vi "9T position.vi"(11 "Instrument":T1={"325 Resource "="GPIB0::13::INSTR", "Input (0:A) 325"=0, "Heater Output (1:1) 325"=1, "340 Resource"="GPIB0::14::INSTR", "Input (0:A) 340"=0, "Loop (0: 1)"=0, "Input (0:B) 340"=1, "Loop (1: 1)"=0, "340 Status"=refnum, "Instrument Type"=enum."PPMS-Rotate", "quantum design"=refnum, "semaphore 325"=refnum, "TCP master instance"=refnum, "M24C Resource"="GPIB0::24::INSTR", "4G supply"="GPIB0::24::INSTR", "Temp Status 24C"=refnum, "Temp"=refnum, "9T信号"=refnum, "limit"={"Field limit"=0.0, "Field rate limit"=0.0, "Temp limit"=0.0, "Temp low limit"=0.0, "Temp rate limit "=0.0}, "4g supply status"=refnum, "vi路径"="", "in-plane"="", "out-plane"="", "in-plane signal"=FALSE, "out-plane signal"=FALSE, "in plane 信号"=refnum, "pzt volt"=refnum, "Aborting"=refnum, "数据文件"=refnum, "warning"=refnum, "750 visa"="", "750 rotate"="", "335 Status 2"=refnum, "335 Resource "="GPIB0::24::INSTR", "Input (0:A) 335"=0, "Input (0:B) 335"=1, "Heater Output (1:1) 335"=1, "semaphore 340"=refnum, "semaphore 335"=refnum, "325 Status"=refnum, "semaphore 750"=refnum, "750 field status"=refnum, "camg 振荡状态"=refnum, "列表框"=refnum, "编辑列表框？"=refnum, "camg Rate"=refnum, "行数"=refnum, "TM620"="TCPIP0::192.168.1.5::4266::SOCKET"} {"Loop (1: 1)" items=["1"=1, "2"=2]; "Loop (0: 1)" items=["1"=1, "2"=2]; "Input (0:B) 340" items=["A", "B", "C", "D"]; "Heater Output (1:1) 335" items=["1"=1, "2"=2]; "Input (0:B) 335" items=["A", "B"]; "Input (0:A) 335" items=["A", "B"]; "Heater Output (1:1) 325" items=["1"=1, "2"=2]; "Input (0:A) 325" items=["A", "B"]; "Input (0:A) 340" items=["1"=1, "2"=2]}) -> (2 "in plane":dbl, 3 "out plane":dbl)   [LabVIEW 2019, in "9T cmag.lvlib"]
uses:
  9T cmag.lvlib
  ctl/Instrument.ctl
  <vilib>/NI/Modbus Library/API/Master/Modbus Master.lvclass
  ctl/335 state.ctl
  ctl/Instrument Type.ctl
  C:/Users/fuyang/Desktop/postdoctor/labview/labview-measure/lib/QDInstrument.dll
  lib/QDInstrument.dll
  ctl/limit.ctl
  ctl/9T mag field stauts.ctl
  ctl/warning.ctl
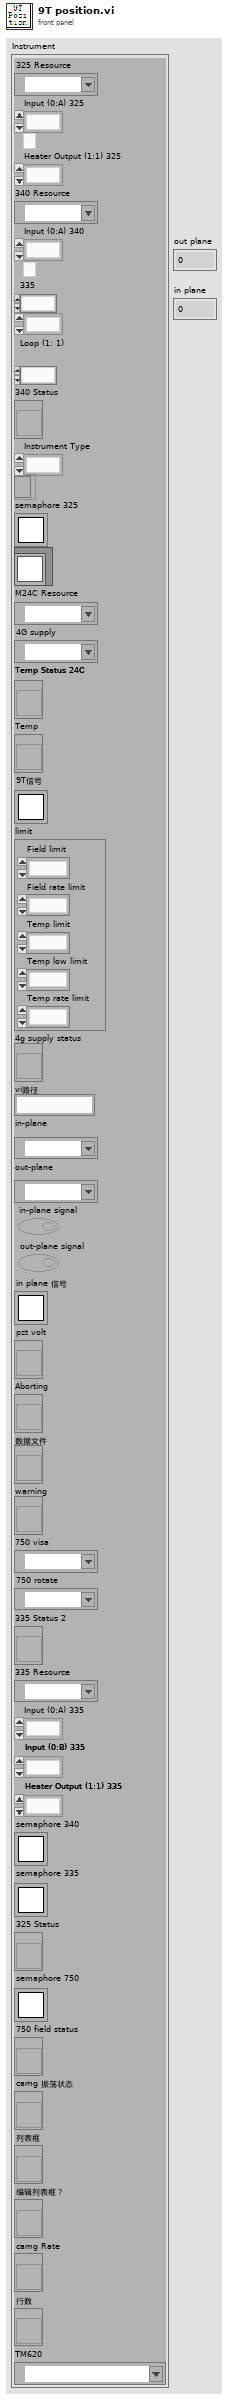
[diagram p1: front panel]
types:
  T1 = typedef "Instrument.ctl" = cluster{"325 Resource ":refnum<visa-resource-name>, "Input (0:A) 325":u16, "Heater Output (1:1) 325":u16, "340 Resource":refnum<visa-resource-name>, "Input (0:A) 340":u16, "Loop (0: 1)":u16, "Input (0:B) 340":u16, "Loop (1: 1)":u16, "340 Status":refnum<vi>, "Instrument Type":T2, "quantum design":refnum<k24>, "semaphore 325":T3, "TCP master instance":refnum<class "Modbus Master.lvclass">, "M24C Resource":refnum<visa-resource-name>, "4G supply":refnum<visa-resource-name>, "Temp Status 24C":refnum<vi>, "Temp":refnum<vi>, "9T信号":T3, "limit":T4, "4g supply status":refnum<vi>, "vi路径":string, "in-plane":refnum<visa-resource-name>, "out-plane":refnum<visa-resource-name>, "in-plane signal":bool, "out-plane signal":bool, "in plane 信号":T3, "pzt volt":refnum<vi>, "Aborting":refnum<vi>, "数据文件":refnum<vi>, "warning":refnum<vi>, "750 visa":refnum<visa-resource-name>, "750 rotate":refnum<visa-resource-name>, "335 Status 2":refnum<vi>, "335 Resource ":refnum<visa-resource-name>, "Input (0:A) 335":u16, "Input (0:B) 335":u16, "Heater Output (1:1) 335":u16, "semaphore 340":T3, "semaphore 335":T3, "325 Status":refnum<vi>, "semaphore 750":T3, "750 field status":refnum<vi>, "camg 振荡状态":refnum<vi>, "列表框":refnum<vi>, "编辑列表框？":refnum<vi>, "camg Rate":refnum<vi>, "行数":refnum<vi>, "TM620":refnum<visa-resource-name>}
  T2 = typedef "Instrument Type.ctl" = enum16{"PPMS", "VersaLab", "DynaCool", "SVSM", "PPMS-Rotate", "Lakeshore335", "lengtou2", "9T mag old", "9T cmag", "9T cmag DAC", "9T cmag rotate", "test"}
  T3 = typedef "Semaphore RefNum" = refnum<k1>
  T4 = typedef "limit.ctl" = cluster{"Field limit":dbl, "Field rate limit":dbl, "Temp limit":dbl, "Temp low limit":dbl, "Temp rate limit ":dbl}
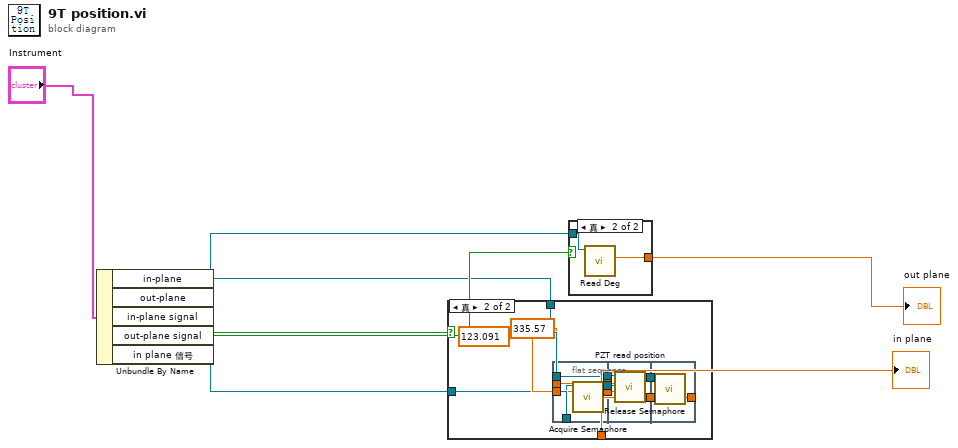
[diagram p0: block diagram]
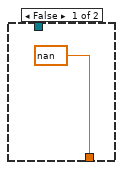
[diagram p2: hidden frame]
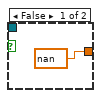
[diagram p3: hidden frame]
diagram:
  n1 = Unbundle By Name("Instrument") -> ("in-plane"=w5:refnum<visa-resource-name>, "out-plane"=w6:refnum<visa-resource-name>, "in-plane signal"=w7:bool, "out-plane signal"=w8:bool, "in plane 信号"=w1:T3)
  n2 = case shown="真" w7 {
    tunnel: w5 -> [_ w20]
    tunnel: [nan w19] -> w3
    tunnel: w1 -> [_ w12]
    frame False {
    }
    frame True {
      n3 = flat-sequence {
        tunnel: 123.091 ("Origin") -> [w23]
        tunnel: 335.57 ("Range") -> [w24]
        tunnel: w20 -> [w25]
        tunnel: [w25] -> w16
        tunnel: [w24] -> w15
        tunnel: [w23] -> w14
        tunnel: w12 -> [w22]
        tunnel: [w21] -> w11
        tunnel: w16 -> [w30]
        tunnel: w15 -> [w28]
        tunnel: w14 -> [w27]
        tunnel: [w29] -> w13
        tunnel: w11 -> [w26]
        tunnel: [w26] -> w10
        tunnel: [w32] -> w19
        tunnel: w13 -> [w32]
        tunnel: w10 -> [w31]
        frame #0 {
          n4 = call <vilib>:"Acquire Semaphore.vi"("semaphore"=w22) -> ("semaphore out"=w21:T3)  [unwired: 4 in, 2 out]
        }
        frame #1 {
          n5 = call "PZT read position.vi"("Origin"=w27, "Range"=w28, "VISA resource name"=w30) -> ("Current Position （mm  /  °）"=w29:dbl)  [unwired: 1 in, 2 out]
        }
        frame #2 {
          n6 = call <vilib>:"Release Semaphore.vi"("semaphore"=w31) -> ()  [unwired: 5 in, 2 out]
        }
      }
    }
  }
  "in plane" <- w3
  n7 = case shown="真" w8 {
    tunnel: w6 -> [_ w35]
    tunnel: [nan w34] -> w2
    frame False {
    }
    frame True {
      n8 = call "Read Deg.vi"("VISA resource name out"=w35) -> ("角度"=w34:dbl)  [unwired: 8 in, 2 out]
    }
  }
  "out plane" <- w2
